vi "Read Measured Values.vi"(8 "error in (no error)":errorcluster, 11 "VGC in":refnum<class "PL Inficon VGC.lvclass">) -> (0 "error out":errorcluster, 2 "measured values":cluster{"status":u16, "value":dbl}[](array[cluster]) {"status" items=["data ok", "underrange", "overrange", "sensor error", "sensor off", "no sensor", "identification error", "error BPG, HPG, BCG"]; "value" format="%#_4p"}, 3 "VGC out":refnum<class "PL Inficon VGC.lvclass">)   [LabVIEW 2015, in "PL Inficon VGC.lvclass"]
doc: "Reads measured values."
uses:
  PL Inficon VGC.lvclass
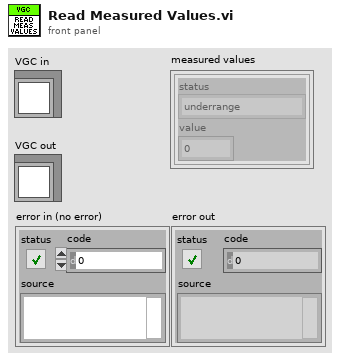
[diagram p1: front panel]
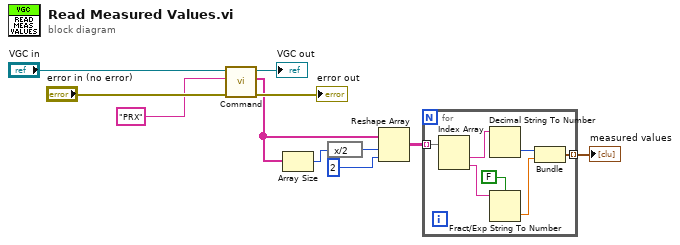
[diagram p0: block diagram]
diagram:
  n1 = call "Command.vi"("error in (no error)"="error in (no error)", "command"="PRX", "VGC in"="VGC in") -> ("error out"=→"error out":errorcluster, "response data"=w6:string[], "VGC out"=→"VGC out":refnum<class "PL Inficon VGC.lvclass">)  [unwired: 6 in]
  n2 = Array Size(array=w6) -> (size(s)=w5:i32)
  n3 = expression code="x/2"(w5) -> (w4:i32)
  n4 = Reshape Array(w6, w4, 2 ("dimension size")) -> (w2:string[][])
  n5 = for {
    tunnel: w2 -> [w18] mode=indexing
    tunnel: [w12] -> w1 mode=indexing
    n6 = Index Array(array=w18) -> (element #1=w15:string, element #2=w16:string)  [unwired: 2 in]
    n7 = Decimal String To Number(string=w15) -> (number=w14:i32)  [unwired: 2 in, 1 out]
    n8 = Fract/Exp String To Number(use system decimal point (T)=FALSE, string=w16) -> (number=w13:dbl)  [unwired: 2 in, 1 out]
    n9 = Bundle(w14, w13) -> (w12:cluster{i32, dbl})  [unwired: 1 in]
  }
  "measured values" <- w1
